vi "Random String.vi"(4 "Length":i32) -> (1 "ASCII":string)   [LabVIEW 2013]
uses:
  <userlib>/_OpenG.lib/numeric/numeric.llb/Random Number Within Range - I32__ogtk.vi
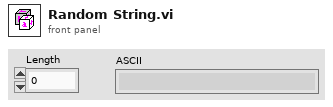
[diagram p1: front panel]
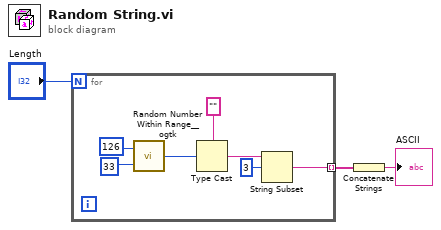
[diagram p0: block diagram]
diagram:
  n1 = for {
    N: "Length" -> [_]
    tunnel: [w4] -> w3 mode=indexing
    n2 = call-poly <userlib>:"Random Number Within Range__ogtk.vi"("High"=126, "Low"=33) -> ("Random Number"=w7:i32)  [unwired: 3 in]
    n3 = Type Cast(type="" ("string"), x=w7) -> (*(type *) &x=w6:string)
    n4 = String Subset(string=w6, offset (0)=3) -> (substring=w4:string)  [unwired: 1 in]
  }
  n5 = Concatenate Strings(w3) -> (→"ASCII":string)
